vi "Autonomous Independent.vi"() -> ()   [LabVIEW 2020]
doc: "This VI is called when autonomous begins, and will automatically be terminated when autonomous ends. You can carry out timed or sensor driven robot movement independently without needing to return to the caller."
uses:
  <vilib>/Rock Robotics/WPI/RobotDrive/WPI_RobotDriveArcadeDrive_Standard(NoSaturation).vi
  <vilib>/Rock Robotics/Network Tables/NT Write Numeric Array.vi
  <vilib>/addons/control/pid/NI_PID_pid.lvlib
  <vilib>/addons/control/pid/pid.llb/PID (DBL).vi
  <vilib>/addons/control/pid/pid.llb/PID Output Rate Limiter (DBL).vi
  <vilib>/Rock Robotics/Network Tables/NT Read String.vi
  Color-Sensor-v3-Examples-master/LabVIEW/Color Match/Global 1.vi
panel:
  in  "Time           Distance     Angle      Gain             Reset":dbl[][](array[numeric])=[[0.0, 0.0, 0.0, 0.0, 0.0], [5.0, 0.0, 0.0, 0.0, 0.0], [5.1, 72.0, 0.0, 1.0, 0.0], [10.0, 72.0, 0.0, 1.0, 0.0], [10.1, 72.0, 0.0, 1.0, 0.0], [15.0, 72.0, 0.0, 1.0, 0.0], [15.1, 72.0, 180.0, 0.0, 0.0], [20.0, 72.0, 180.0, 0.0, 0.0], [20.1, 144.0, 180.0, 1.0, 0.0], [25.0, 144.0, 180.0, 1.0, 0.0], [25.1, 144.0, 360.0, 0.0, 0.0], [30.0, 144.0, 360.0, 0.0, 0.0], [30.1, 216.0, 360.0, 1.0, 0.0], [35.0, 216.0, 360.0, 1.0, 0.0], [50.0, 216.0, 360.0, 1.0, 0.0], [0.0, 0.0, 0.0, 0.0, 0.0], [0.0, 0.0, 0.0, 0.0, 0.0], [0.0, 0.0, 0.0, 0.0, 0.0], [0.0, 0.0, 0.0, 0.0, 0.0], [0.0, 0.0, 0.0, -1.0, 0.0]]
  in  "Wheelbase (in)":dbl=26.0
  in  "Wheel Diameter (in)":dbl=6.0
  in  "Stop":bool
  out "Left Motor\nCommand":dbl(knob)=0.05112453377819276 scale=-1.0..1.0
  out "Right Motor\nCommand":dbl(knob)=0.044089840607117875 scale=-1.0..1.0
  out "Left Target":dbl=72.0
  out "Chart":T1(graph)={"Distance (in)"=73.72400612920396, 72.0, "Distance (in)"=73.89025921243193, 72.0}
  out "Right Target":dbl=72.0
  out "Angles":cluster{dbl, "Z Axis (deg)":dbl}(graph)={0.0, "Z Axis (deg)"=-6.362208713333332}
  out "Angle":dbl=-6.362208713333332
  out "Left Distance":dbl=73.72400612920396
  out "Right Distance":dbl=73.89025921243193
  out "Encoder\nReset":cluster{dbl}(graph)
  out "Gain Cmd":dbl=1.0
  in  "PID Gains for Straight":T2={"Prop gain (Kc)"=0.015, "Int time (Ti)"=0.09, "Deriv time (Td)"=0.005} {"Deriv time (Td)" format="%.4f"; "Int time (Ti)" format="%.4f"; "Prop gain (Kc)" format="%.4f"}
  in  "PID Gains For Turning":T2={"Prop gain (Kc)"=0.032, "Int time (Ti)"=0.027, "Deriv time (Td)"=0.004} {"Deriv time (Td)" format="%.4f"; "Int time (Ti)" format="%.4f"; "Prop gain (Kc)" format="%.4f"}
  out "s? t:f":T2={"Prop gain (Kc)"=0.015, "Int time (Ti)"=0.08, "Deriv time (Td)"=0.005}
  out "Reset":dbl
  in  "right output rate (EGU/min)":dbl=100.0 format="%.2f"
  in  "left output rate (EGU/min)":dbl=100.0 format="%.2f"
  out "Current Movement, for debugging":T3 {"Y Joystick Value" scale=1.0..-1.0; "X Joystick Value" scale=-1.0..1.0}
  in  "Array of robot movements":T4(array[cluster])=[{"X Joystick Value"=0.39393939393939403, "Y Joystick Value"=0.0, "Delay (sec)"=1.0, "Movement Name"="turn"}, {"X Joystick Value"=-0.3737373737373737, "Y Joystick Value"=0.0, "Delay (sec)"=1.0, "Movement Name"="turn back"}] {"Y Joystick Value" scale=1.0..-1.0; "X Joystick Value" scale=-1.0..1.0}
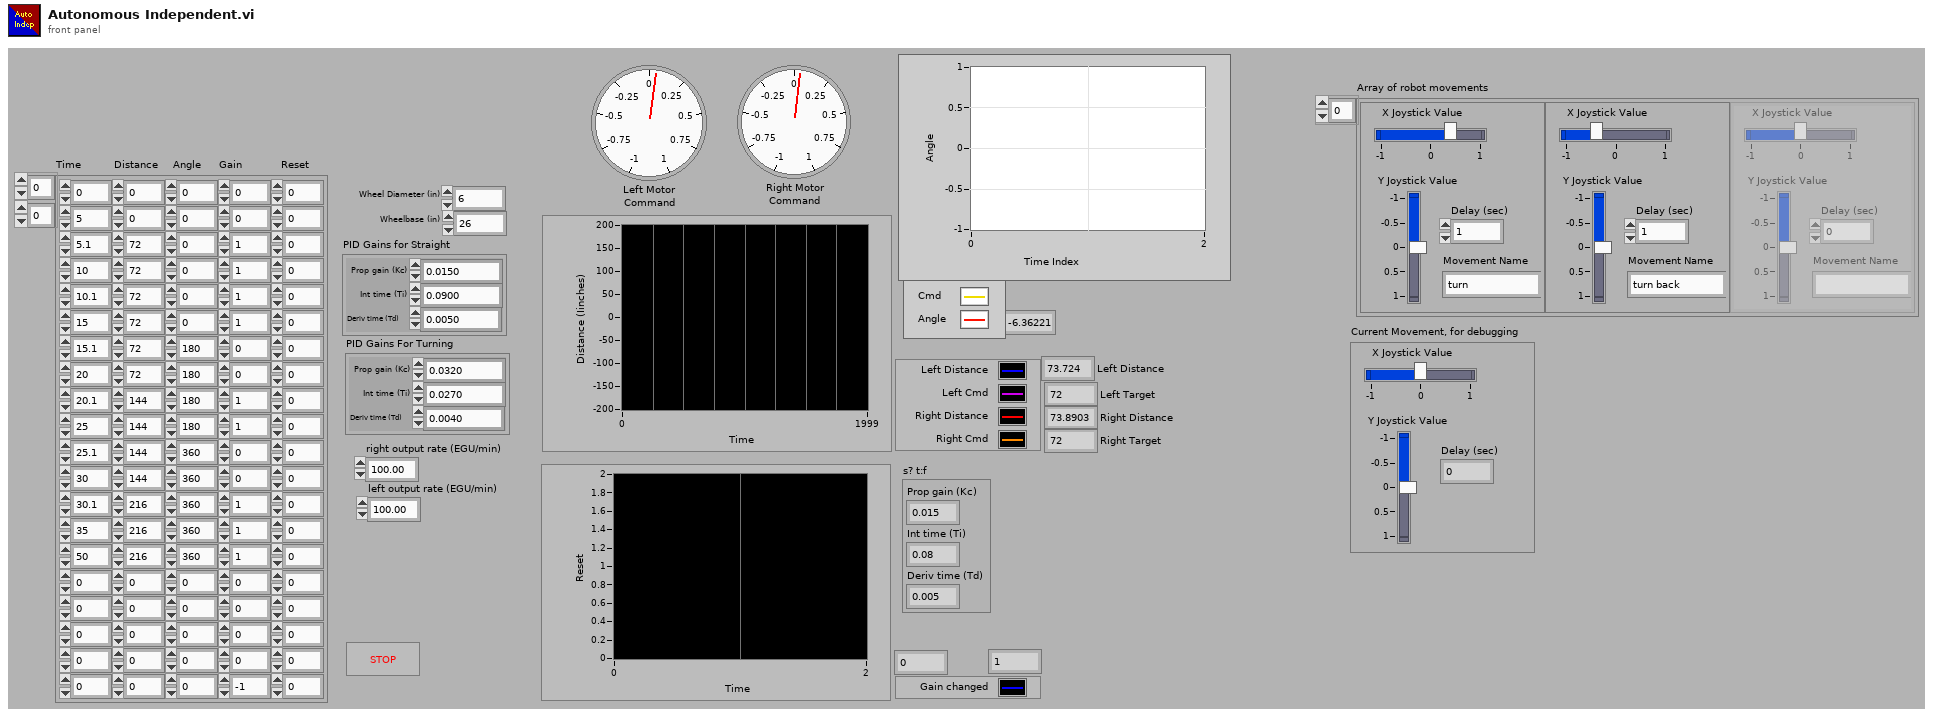
[diagram p1: front panel]
types:
  T1 = cluster{"Distance (in)":dbl, dbl, "Distance (in)":dbl, dbl}
  T2 = cluster{"Prop gain (Kc)":dbl, "Int time (Ti)":dbl, "Deriv time (Td)":dbl}
  T3 = cluster{"X Joystick Value":dbl, "Y Joystick Value":dbl, "Delay (sec)":dbl, "Movement Name":string}
  T4 = cluster{"X Joystick Value":dbl, "Y Joystick Value":dbl, "Delay (sec)":dbl, "Movement Name":string}[]
  T5 = typedef "WPI_JoystickDevRef.ctl" = cluster{"Device":T6}
  T6 = typedef "WPI_JoystickDeviceEnum.ctl" = enum16{"USB 0", "USB 1", "USB 2", "USB 3", "USB 4", "USB 5"}
  T7 = typedef "WPI_EncoderDevRef.ctl" = cluster{"DevStatus":errorcluster, "EncoderIndex":T8, "CounterIndex":T9, "DistancePerCount":dbl, "Decoding Type":T10}
  T8 = typedef "FPGA_EncoderIdx.ctl" = enum8{"Enc 0", "Enc 1", "Enc 2", "Enc 3", "Enc 4", "Enc 5", "Enc 6", "Enc 7", "Invalid"}
  T9 = typedef "FPGA_CounterCtrSystemIndex.ctl" = enum8{"Ctr 0", "Ctr 1", "Ctr 2", "Ctr 3", "Ctr 4", "Ctr 5", "Ctr 6", "Ctr 7", "Invalid"}
  T10 = typedef "WPI_EncoderType.ctl" = enum16{"1x", "2x", "4x"}
  T11 = typedef "WPI_MotorControlDeviceRef.ctl" = cluster{"DeviceStatus":errorcluster, "Type":T12, "PWM":cluster{"PWM Channel":T13, "DeadBand":T14}, "CAN":cluster{"Device Number":u8, "SetOutput VI Ref":variant, "GetOutput VI Ref":variant, "Enable VI Ref":variant, "Disable VI Ref":variant, "Data":variant}, "Invert":bool, "DIO PWM":cluster{"PWM \"Enable\" Channel":T13, "DIOChannel":T15, "PWM Rate":dbl}}
  T12 = typedef "WPI_MotorControlType.ctl" = enum16{"PWM", "CAN", "DIO PWM"}
  T13 = typedef "FPGA_DIOPWMChannel.ctl" = enum8{"PWM 0", "PWM 1", "PWM 2", "PWM 3", "PWM 4", "PWM 5", "PWM 6", "PWM 7", "PWM 8", "PWM 9", "PWM MXP 0", "PWM MXP 1", "PWM MXP 2", "PWM MXP 3", "PWM MXP 4", "PWM MXP 5", "PWM MXP 6", "PWM MXP 7", "PWM MXP 8", "PWM MXP 9", "Invalid"}
  T14 = typedef "WPI_PWMDeadband.ctl" = cluster{"Name":string, "maxPositivePwm":i32, "minPositivePwm":i32, "centerPwm":i32, "maxNegativePwm":i32, "minNegativePwm":i32, "angularRange":u16}
  T15 = typedef "FPGA_DIOChannel.ctl" = enum8{"DIO 0", "DIO 1", "DIO 2", "DIO 3", "DIO 4", "DIO 5", "DIO 6", "DIO 7", "DIO 8", "DIO 9", "DIO MXP 0", "DIO MXP 1", "DIO MXP 2", "DIO MXP 3", "DIO MXP 4", "DIO MXP 5", "DIO MXP 6", "DIO MXP 7", "DIO MXP 8", "DIO MXP 9", "DIO MXP 10", "DIO MXP 11", "DIO MXP 12", "DIO MXP 13", "DIO MXP 14", "DIO MXP 15", "SPI Port CS1", "SPI Port CS2", "SPI Port CS3", "SPI Port MISO", "SPI Port MOSI", "Invalid"}
  T16 = typedef "WPI_I2CDevRef.ctl" = cluster{"DevStatus":errorcluster, "Device Address":u8, "Handle":i32, "I2C Bus":T17}
  T17 = typedef "i2c_bus.ctl" = enum16{"I2C On-Board", "I2C MXP", "Invalid"}
  T18 = cluster{"Gyro X":dbl, "Gyro Y":dbl, "Gyro Z":dbl}
  T19 = cluster{"Left Side Angular Velocity":dbl, "Left Side Revs":dbl, "Left Side Distance (in)":dbl, "Left Side Angle (Angle)":dbl}
  T20 = cluster{"Right Side Angular Velocity":dbl, "Right Side Revs":dbl, "Right Side Distance":dbl, "Right Side Angle (deg)":dbl}
  T21 = cluster{"X Axis (deg)":dbl, "Y Axis (deg)":dbl, "Z Axis (deg)":dbl}
  T22 = cluster{"Left Side Distance (in)":dbl, "Left Distance Target":dbl, "Right Side Distance":dbl, "Right Distance Target":dbl}
  T23 = typedef "WPI_RobotDriveDevRef.ctl" = cluster{"DevStatus":errorcluster, "Motors[]":T11[], "Square Inputs":bool, "Max Output":dbl}
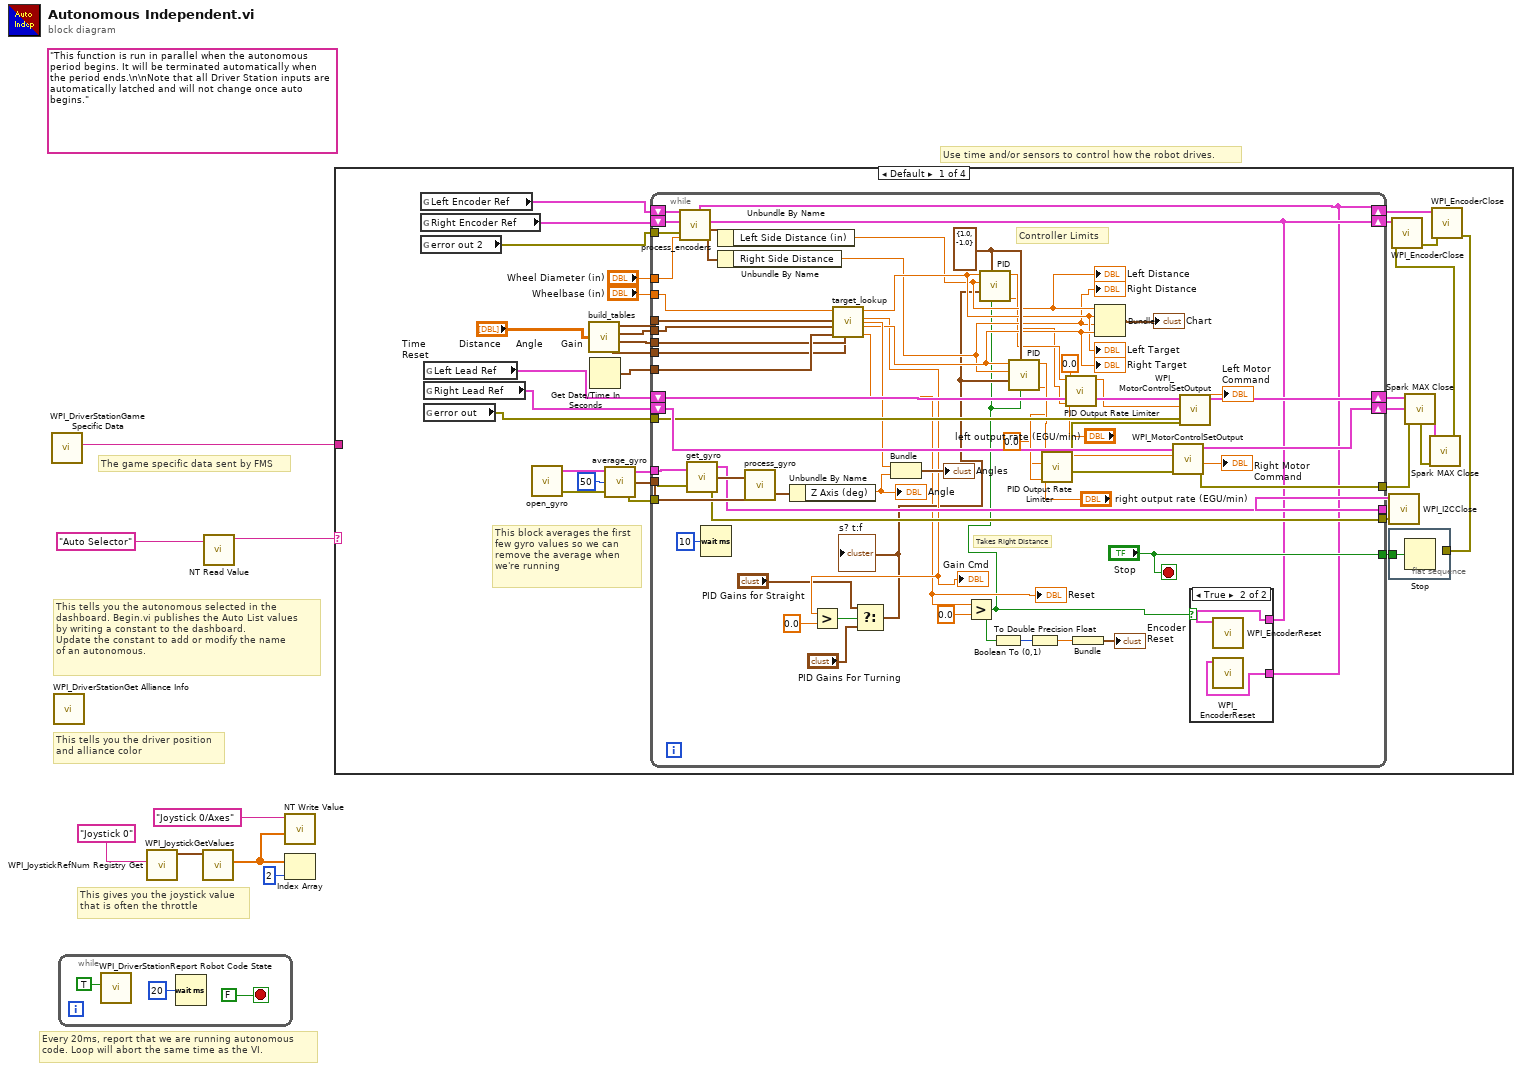
[diagram p0: block diagram]
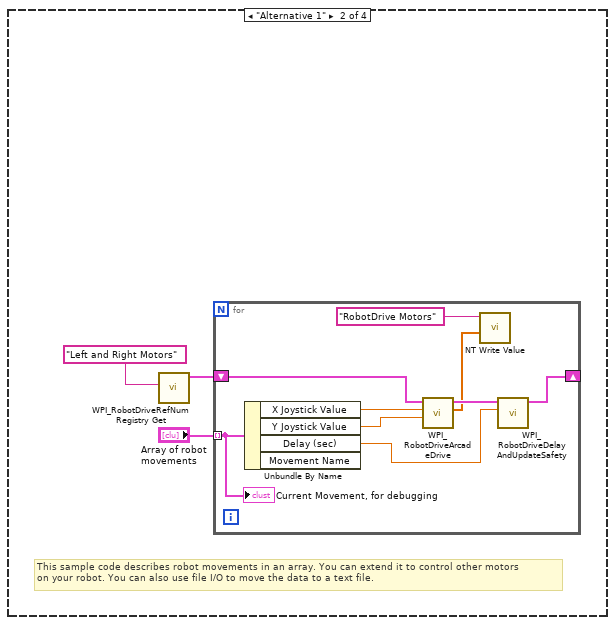
[diagram p3: hidden frame]
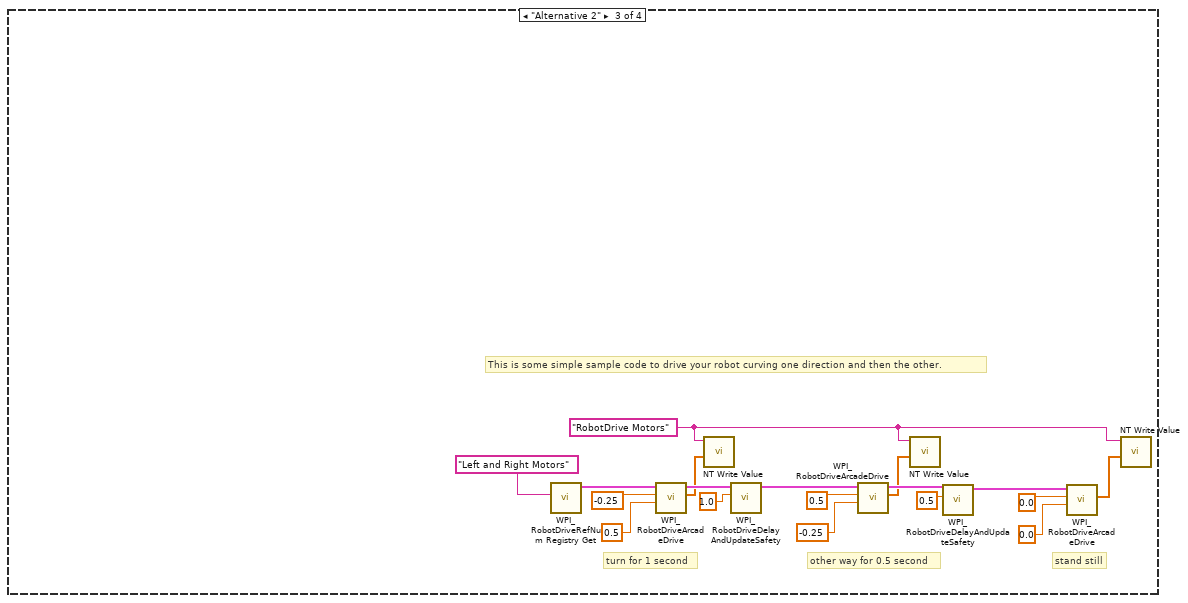
[diagram p4: hidden frame]
diagram:
  (unwired) "This function is run in parallel when the autonomous period begins. It will be terminated automatically when the period ends.\n\nNote that all Driver Station inputs are automatically latched and will not change once auto begins."
  # "The game specific data sent by FMS"
  # "This tells you the autonomous selected in the \ndashboard. Begin.vi publishes the Auto List values\nby writing a constant to the dashboard.\nUpdate the constant to add or modify the name\nof an autonomous."
  # "Every 20ms, report that we are running autonomous\ncode. Loop will abort the same time as the VI."
  # "This gives you the joystick value\nthat is often the throttle"
  # "Use time and/or sensors to control how the robot drives."
  # "This tells you the driver position\nand alliance color"
  n1 = call <vilib>:"WPI_DriverStationGame Specific Data.vi"() -> ("Game Specific Data"=w1:string)  [unwired: 11 in]
  n2 = call <vilib>:"WPI_DriverStationGet Alliance Info.vi"() -> ()  [unwired: 12 out]
  n3 = while {
    stop <- FALSE stop-if-true
    n4 = call <vilib>:"WPI_DriverStationReport Robot Code State.vi"("Autonomous"=TRUE) -> ()  [unwired: 10 in, 1 out]
    n5 = Wait (ms)(milliseconds to wait=u32 20) -> ()  [unwired: 1 out]
  }
  n6 = call <vilib>:"WPI_JoystickRefNum Registry Get.vi"("refnum name"="Joystick 0") -> ("JoystickDevRef"=w7:T5)  [unwired: 1 in, 9 out]
  n7 = call <vilib>:"WPI_JoystickGetValues.vi"("JoystickDevRef"=w7) -> ("Axes"=w3:dbl[])  [unwired: 6 in, 4 out]
  n8 = call-poly <vilib>:"NT Read Value.vi"("Name"="Auto Selector") -> ("String"=w4:string)  [unwired: 9 in, 1 out]
  n9 = call-poly <vilib>:"NT Write Value.vi"("Numeric Array"=w3, "Name"="Joystick 0/Axes") -> ()  [unwired: 9 in, 1 out]
  n10 = Index Array(array=w3, index=2) -> ()  [unwired: 1 out]
  n11 = case shown="Default" w4 {
    tunnel: w1 -> [_ _ _ _]
    frame Default {
      # "This block averages the first few gyro values so we can remove the average when we're running"
      n12 = global read "Global 1.vi" "Left Encoder Ref"() -> (w14:T7)
      n13 = global read "Global 1.vi" "Right Encoder Ref"() -> (w13:T7)
      n14 = global read "Global 1.vi" "error out 2"() -> (w12:errorcluster)
      n15 = global read "Global 1.vi" "Left Lead Ref"() -> (w17:T11)
      n16 = global read "Global 1.vi" "Right Lead Ref"() -> (w16:T11)
      n17 = global read "Global 1.vi" "error out"() -> (w15:errorcluster)
      n18 = call "open_gyro.vi"() -> ("error out"=w31:errorcluster, "I2CDevRef"=w32:T16)  [unwired: 1 in]
      n19 = call "build_tables.vi"("Target Table"="Time           Distance     Angle      Gain             Reset") -> ("Distance Table"=w22:cluster{"Numeric":dbl, "Numeric":dbl}[], "Angle Table"=w21:cluster{"Numeric":dbl, "Numeric":dbl}[], "Gain Table"=w19:cluster{"Numeric":dbl, "Numeric":dbl}[], "Encoder Table"=w18:cluster{"Numeric":dbl, "Numeric":dbl}[])
      n20 = Get Date/Time In Seconds() -> (seconds since 1Jan1904=w33:timestamp)
      n21 = call "average_gyro.vi"("error in"=w31, "Times to Avg"=50, "I2CDevRef in"=w32) -> ("error out"=w28:errorcluster, "Average Raw Gyro Values"=w30:T18, "I2CDevRef Out"=w29:T16)
      n22 = while {
        shift-right: [w68] -> w43
        shift-left: w14 -> [w90]
        tunnel: ["Stop"] -> w42
        tunnel: "Wheel Diameter (in)" -> [w87]
        shift-right: [w71] -> w40
        shift-left: w13 -> [w88]
        shift-right: [w104] -> w37
        shift-left: w17 -> [w100]
        shift-right: [w103] -> w36
        shift-left: w16 -> [w105]
        tunnel: [w82] -> w38
        tunnel: w15 -> [w84]
        tunnel: "Wheelbase (in)" -> [w81]
        tunnel: w33 -> [w79]
        tunnel: w22 -> [w80]
        tunnel: w30 -> [w96]
        tunnel: w29 -> [w95]
        tunnel: w28 -> [w94]
        tunnel: [w77] -> w27
        tunnel: [w93] -> w26
        tunnel: w12 -> [w89]
        tunnel: w21 -> [w70]
        tunnel: w19 -> [w69]
        tunnel: w18 -> [w58]
        stop <- "Stop" stop-if-true
        w99 = cluster{"output high":dbl, "output low":dbl} {"output high"=1.0, "output low"=-1.0} ("output range")
        # "Takes Right Distance"
        # "Controller Limits"
        n23 = call "process_encoders.vi"("Left Encoder Ref In"=w90, "Right Encoder Ref In"=w88, "error in"=w89, "Wheel Diameter (in)"=w87) -> ("Left Encoder Ref Out"=w68:T7, "Right Encoder Ref Out"=w71:T7, "Left Side"=w86:T19, "Right Side"=w76:T20)  [unwired: 1 out]
        n24 = call "get_gyro.vi"("I2CDevRef in"=w95, "error in"=w94) -> ("I2CDevRef Out"=w77:T16, "Gyros"=w97:cluster{dbl, dbl, dbl}, "error out"=w93:errorcluster)
        n25 = Wait (ms)(milliseconds to wait=u32 10) -> ()  [unwired: 1 out]
        n26 = Unbundle By Name(w86) -> ("Left Side Distance (in)"=w73:dbl)
        "Left Distance" <- w73
        n27 = Unbundle By Name(w76) -> ("Right Side Distance"=w72:dbl)
        "Right Distance" <- w72
        n28 = call "process_gyro.vi"("Average Gyro Data"=w96, "Raw Gyro Data"=w97) -> ("Angles"=w92:T21)  [unwired: 1 out]
        n29 = Unbundle By Name(w92) -> ("Z Axis (deg)"=w91:dbl)
        "Angle" <- w91
        n30 = call "target_lookup.vi"("Encoder Table"=w58, "Gain Table 2"=w69, "Initial Time"=w79, "Angle Table"=w70, "Distance Table"=w80, "Wheelbase (in)"=w81) -> ("Encoder Reset"=w56:dbl, "Right Distance Target"=w75:dbl, "Gain Command"=w63:dbl, "Left Distance Target"=w74:dbl, "Angle (deg)"=w78:dbl)
        "Left Target" <- w74
        "Right Target" <- w75
        "Gain Cmd" <- w63
        "Reset" <- w56
        n31 = Greater?(x=w63, y=0.0) -> (0:w64:bool)
        n32 = Select(t="PID Gains for Straight", s=w64, f="PID Gains For Turning") -> (s? t:f=w61:T2)
        "s? t:f" <- w61
        n33 = Bundle("Angle (deg)"=w78, "Z Axis (deg)"=w91) -> (→"Angles":cluster{"Angle (deg)":dbl, "Z Axis (deg)":dbl})  [unwired: 1 in]
        n34 = Greater?(x=w56, y=0.0) -> (0:w55:bool)
        n35 = call-poly <vilib>:"PID.vi"("reinitialize? (F)"=w55, "output range"=w99, "PID gains"=w61, "process variable"=w73, "setpoint"=w74) -> ("dt out (s)"=w47:dbl, "output"=w49:dbl)  [unwired: 5 in]
        n36 = Boolean To (0,1)(Boolean=w55) -> (0, 1=w65:i16)
        n37 = call-poly <vilib>:"PID.vi"("reinitialize? (F)"=w55, "output range"=w99, "PID gains"=w61, "process variable"=w72, "setpoint"=w75) -> ("dt out (s)"=w52:dbl, "output"=w53:dbl)  [unwired: 5 in]
        n38 = To Double Precision Float(number=w65) -> (double precision float=w66:dbl)
        n39 = call-poly <vilib>:"PID Output Rate Limiter.vi"("dt (s)"=w52, "output rate (EGU/min)"="right output rate (EGU/min)", "initial output"=0.0, "input (controller output)"=w53) -> ("output"=w54:dbl)  [unwired: 4 in, 1 out]
        n40 = call-poly <vilib>:"PID Output Rate Limiter.vi"("dt (s)"=w47, "output rate (EGU/min)"="left output rate (EGU/min)", "initial output"=0.0, "input (controller output)"=w49) -> ("output"=w48:dbl)  [unwired: 4 in, 1 out]
        n41 = Bundle(w66) -> (→"Encoder\nReset":cluster{dbl})  [unwired: 1 in]
        n42 = Bundle("Left Side Distance (in)"=w73, "Left Distance Target"=w74, "Right Side Distance"=w72, "Right Distance Target"=w75) -> (→"Chart":T22)  [unwired: 1 in]
        n43 = call <vilib>:"WPI_MotorControlSetOutput.vi"("error in (no error)"=w84, "Output"=w48, "MotorControlDevRef"=w100) -> ("error out"=w83:errorcluster, "Motor Output"=→"Left Motor\nCommand":dbl, "MotorControlDevRef"=w104:T11)  [unwired: 6 in]
        n44 = call <vilib>:"WPI_MotorControlSetOutput.vi"("error in (no error)"=w83, "Output"=w54, "MotorControlDevRef"=w105) -> ("error out"=w82:errorcluster, "Motor Output"=→"Right Motor\nCommand":dbl, "MotorControlDevRef"=w103:T11)  [unwired: 6 in]
        n45 = case shown="True" w55 {
          tunnel: w71 -> [_ w109]
          tunnel: w68 -> [_ w108]
          frame False {
          }
          frame True {
            n46 = call <vilib>:"WPI_EncoderReset.vi"("EncoderDevRef"=w109) -> ()  [unwired: 9 in, 2 out]
            n47 = call <vilib>:"WPI_EncoderReset.vi"("EncoderDevRef"=w108) -> ()  [unwired: 9 in, 2 out]
          }
        }
      }
      n48 = call <vilib>:"WPI_I2CClose.vi"("error in (no error)"=w26, "I2CDevRef"=w27) -> ()  [unwired: 9 in, 1 out]
      n49 = flat-sequence {
        tunnel: w42 -> [w44]
        tunnel: w23 -> [_]
        frame #0 {
          n50 = Stop(stop? (T)=w44) -> ()
        }
      }
      n51 = call <vilib>:"Spark MAX Close.vi"("error in"=w38, "MotorControlDeviceRef"=w37) -> ("error out"=w35:errorcluster)  [unwired: 9 in]
      n52 = call <vilib>:"Spark MAX Close.vi"("error in"=w35, "MotorControlDeviceRef"=w36) -> ("error out"=w24:errorcluster)  [unwired: 9 in]
      n53 = call <vilib>:"WPI_EncoderClose.vi"("error in (no error)"=w24, "EncoderDevRef"=w40) -> ("error out"=w39:errorcluster)  [unwired: 1 in, 8 out]
      n54 = call <vilib>:"WPI_EncoderClose.vi"("error in (no error)"=w39, "EncoderDevRef"=w43) -> ("error out"=w23:errorcluster)  [unwired: 1 in, 8 out]
    }
    frame "Alternative 1" {
      # "This sample code describes robot movements in an array. You can extend it to control other motors\non your robot. You can also use file I/O to move the data to a text file."
      n55 = call <vilib>:"WPI_RobotDriveRefNum Registry Get.vi"("refnum name"="Left and Right Motors") -> ("RobotDriveDevRef"=w111:T23)  [unwired: 1 in, 9 out]
      n56 = for {
        shift-right: [w119] -> _
        shift-left: w111 -> [w120]
        tunnel: "Array of robot movements" -> [w115] mode=indexing
        n57 = Unbundle By Name(w115) -> ("X Joystick Value"=w118:dbl, "Y Joystick Value"=w117:dbl, "Delay (sec)"=w116:dbl)  [unwired: 1 out]
        n58 = call-poly <vilib>:"WPI_RobotDriveArcadeDrive.vi"("Y axis value"=w117, "X axis value"=w118, "RobotDriveDevRef"=w120) -> ("Motor Values"=w113:dbl[], "RobotDriveDevRef"=w121:T23)  [unwired: 1 in, 6 out]
        n59 = call-poly <vilib>:"NT Write Value.vi"("Numeric Array"=w113, "Name"="RobotDrive Motors") -> ()  [unwired: 9 in, 1 out]
        n60 = call <vilib>:"WPI_RobotDriveDelayAndUpdateSafety.vi"("Delay (s)"=w116, "RobotDriveDevRef"=w121) -> ("RobotDriveDevRef 2"=w119:T23)  [unwired: 8 in, 1 out]
        "Current Movement, for debugging" <- w115
      }
    }
    frame "Alternative 2" {
      w123 = "RobotDrive Motors" ("Name")
      # "This is some simple sample code to drive your robot curving one direction and then the other."
      # "stand still"
      # "other way for 0.5 second"
      # "turn for 1 second"
      n61 = call <vilib>:"WPI_RobotDriveRefNum Registry Get.vi"("refnum name"="Left and Right Motors") -> ("RobotDriveDevRef"=w139:T23)  [unwired: 1 in, 9 out]
      n62 = call-poly <vilib>:"WPI_RobotDriveArcadeDrive.vi"("Y axis value"=0.5 ("X axis value"), "X axis value"=-0.25, "RobotDriveDevRef"=w139) -> ("Motor Values"=w122:dbl[], "RobotDriveDevRef"=w132:T23)  [unwired: 1 in, 6 out]
      n63 = call-poly <vilib>:"NT Write Value.vi"("Numeric Array"=w122, "Name"=w123) -> ()  [unwired: 9 in, 1 out]
      n64 = call <vilib>:"WPI_RobotDriveDelayAndUpdateSafety.vi"("Delay (s)"=1.0, "RobotDriveDevRef"=w132) -> ("RobotDriveDevRef 2"=w133:T23)  [unwired: 8 in, 1 out]
      n65 = call-poly <vilib>:"WPI_RobotDriveArcadeDrive.vi"("Y axis value"=-0.25 ("X axis value"), "X axis value"=0.5, "RobotDriveDevRef"=w133) -> ("Motor Values"=w124:dbl[], "RobotDriveDevRef"=w134:T23)  [unwired: 1 in, 6 out]
      n66 = call-poly <vilib>:"NT Write Value.vi"("Numeric Array"=w124, "Name"=w123) -> ()  [unwired: 9 in, 1 out]
      n67 = call <vilib>:"WPI_RobotDriveDelayAndUpdateSafety.vi"("Delay (s)"=0.5, "RobotDriveDevRef"=w134) -> ("RobotDriveDevRef 2"=w135:T23)  [unwired: 8 in, 1 out]
      n68 = call-poly <vilib>:"WPI_RobotDriveArcadeDrive.vi"("Y axis value"=0.0 ("X axis value"), "X axis value"=0.0, "RobotDriveDevRef"=w135) -> ("Motor Values"=w125:dbl[])  [unwired: 1 in, 7 out]
      n69 = call-poly <vilib>:"NT Write Value.vi"("Numeric Array"=w125, "Name"=w123) -> ()  [unwired: 9 in, 1 out]
    }
    frame "Your Turn" {
    }
  }
